vi "MTConnect_data.vi"() -> ()   [LabVIEW 2014]
panel:
  in  "Boolean":bool
  out "size(s)":i32
  out "Array":i32[](array[numeric])
  out "x-y":u32
  in  "Stop Program":bool
  out "CNC Machine":bool
  in  "?":enum32{""}(tab)
  out "Tool position Y":dbl[](graph)
  out "Spindle Speed":dbl[](graph)
  out "Tool position X":dbl[](graph)
  in  "Record speed":bool
  out "Feed rate":dbl[](graph)
  in  "Record feed ratre":bool
  in  "Record linear X":bool
  in  "Record linear Y":bool
  out "Machine status":string
  out "Program name":string
  out "Block of code being executed":string
  out "Machine availability":string
  out "Emergency status":string
  out "Controller mode":string
  in  "Record spindle \n      load":bool
  out "Spindle load":dbl[](graph)
  out "Spindle power consumption":dbl[](graph)
  in  "Record spindle  \n        power":bool
  in  "Record linear Z":bool
  out "Tool position Z":dbl[](graph)
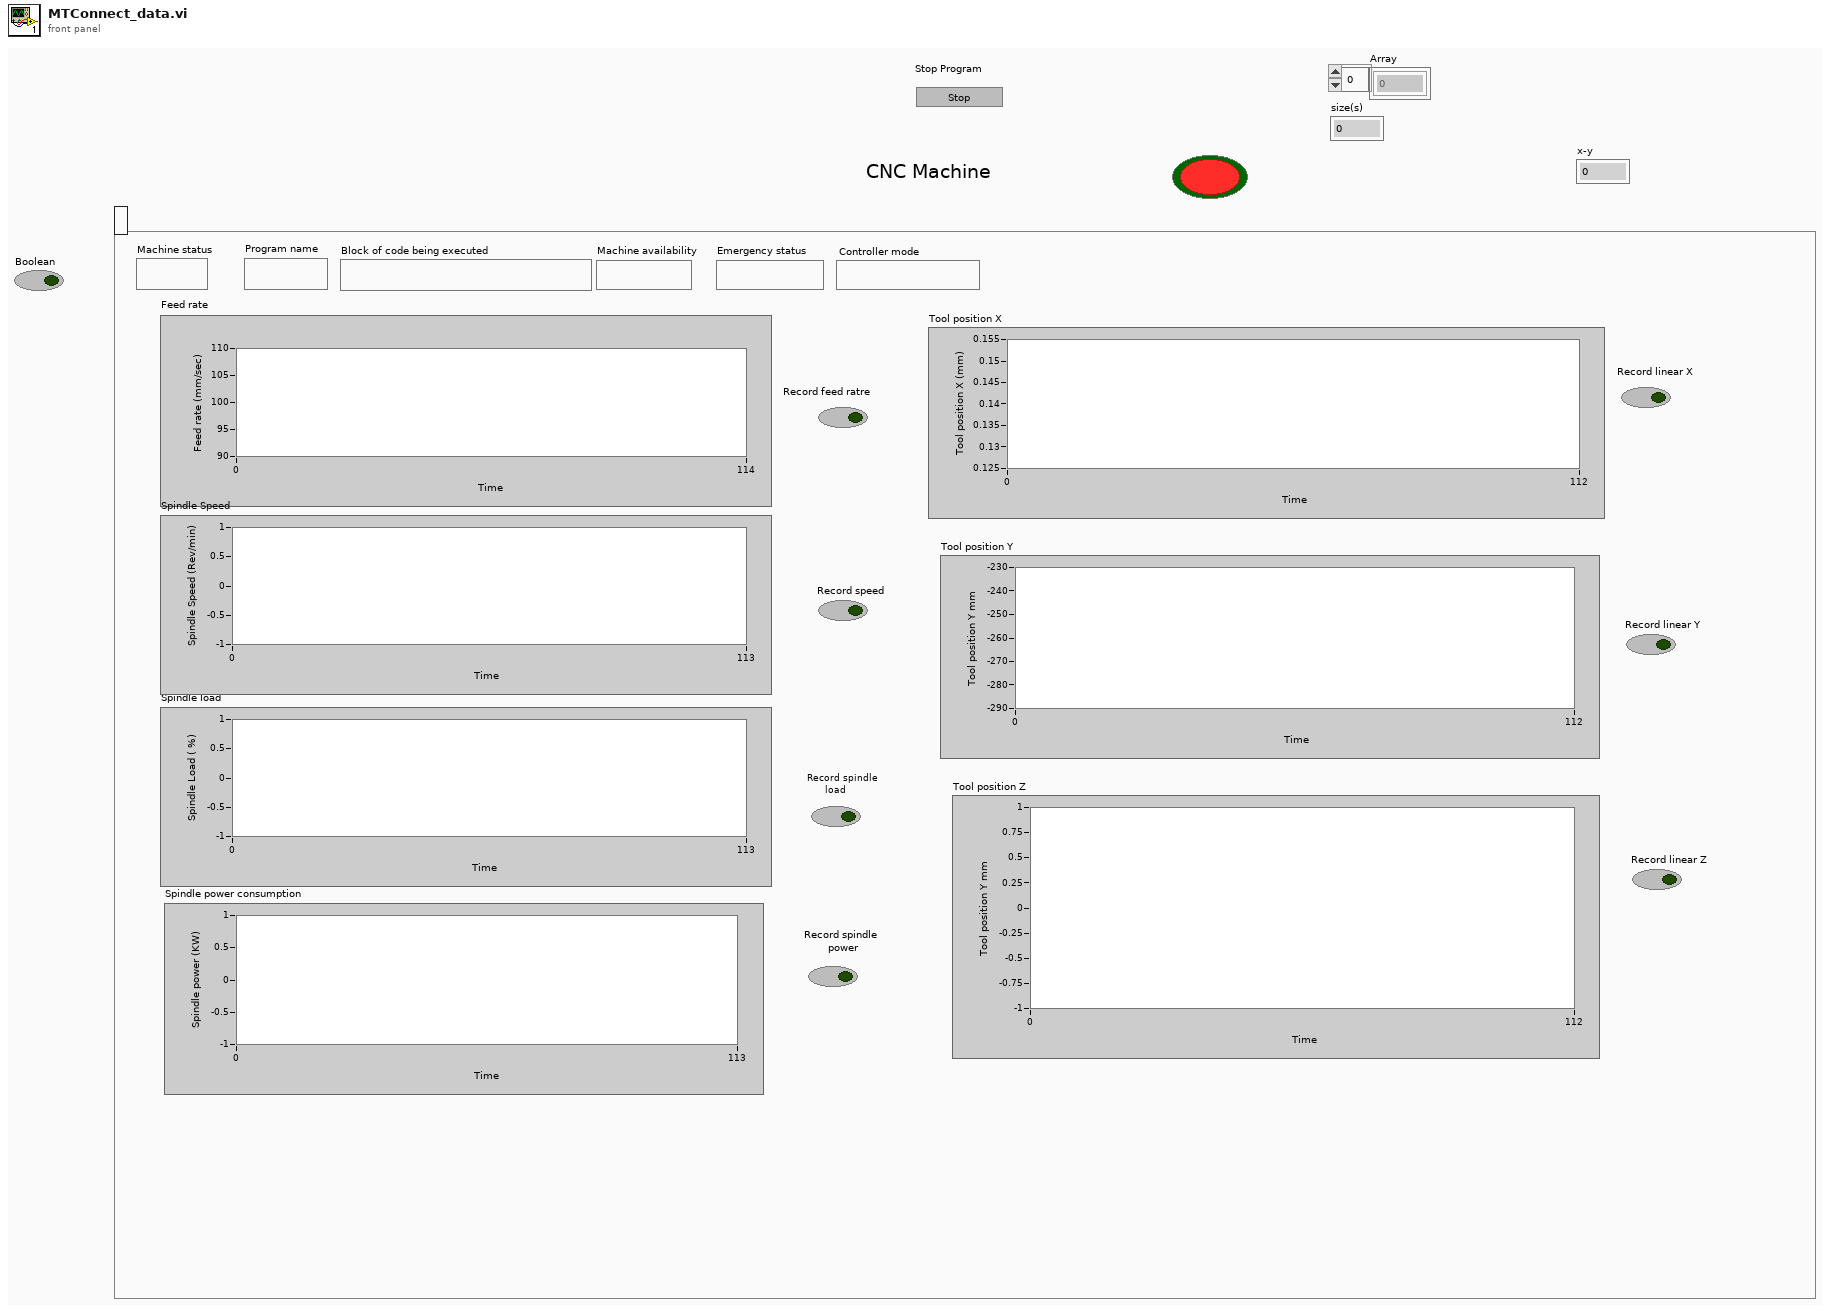
[diagram p1: front panel]
types:
  T1 = cluster{"Program status":string, "Bolck of code being executed":string, "Program name":string, "number":dbl[], "number":dbl[], "number":dbl[], "Boolean":bool}
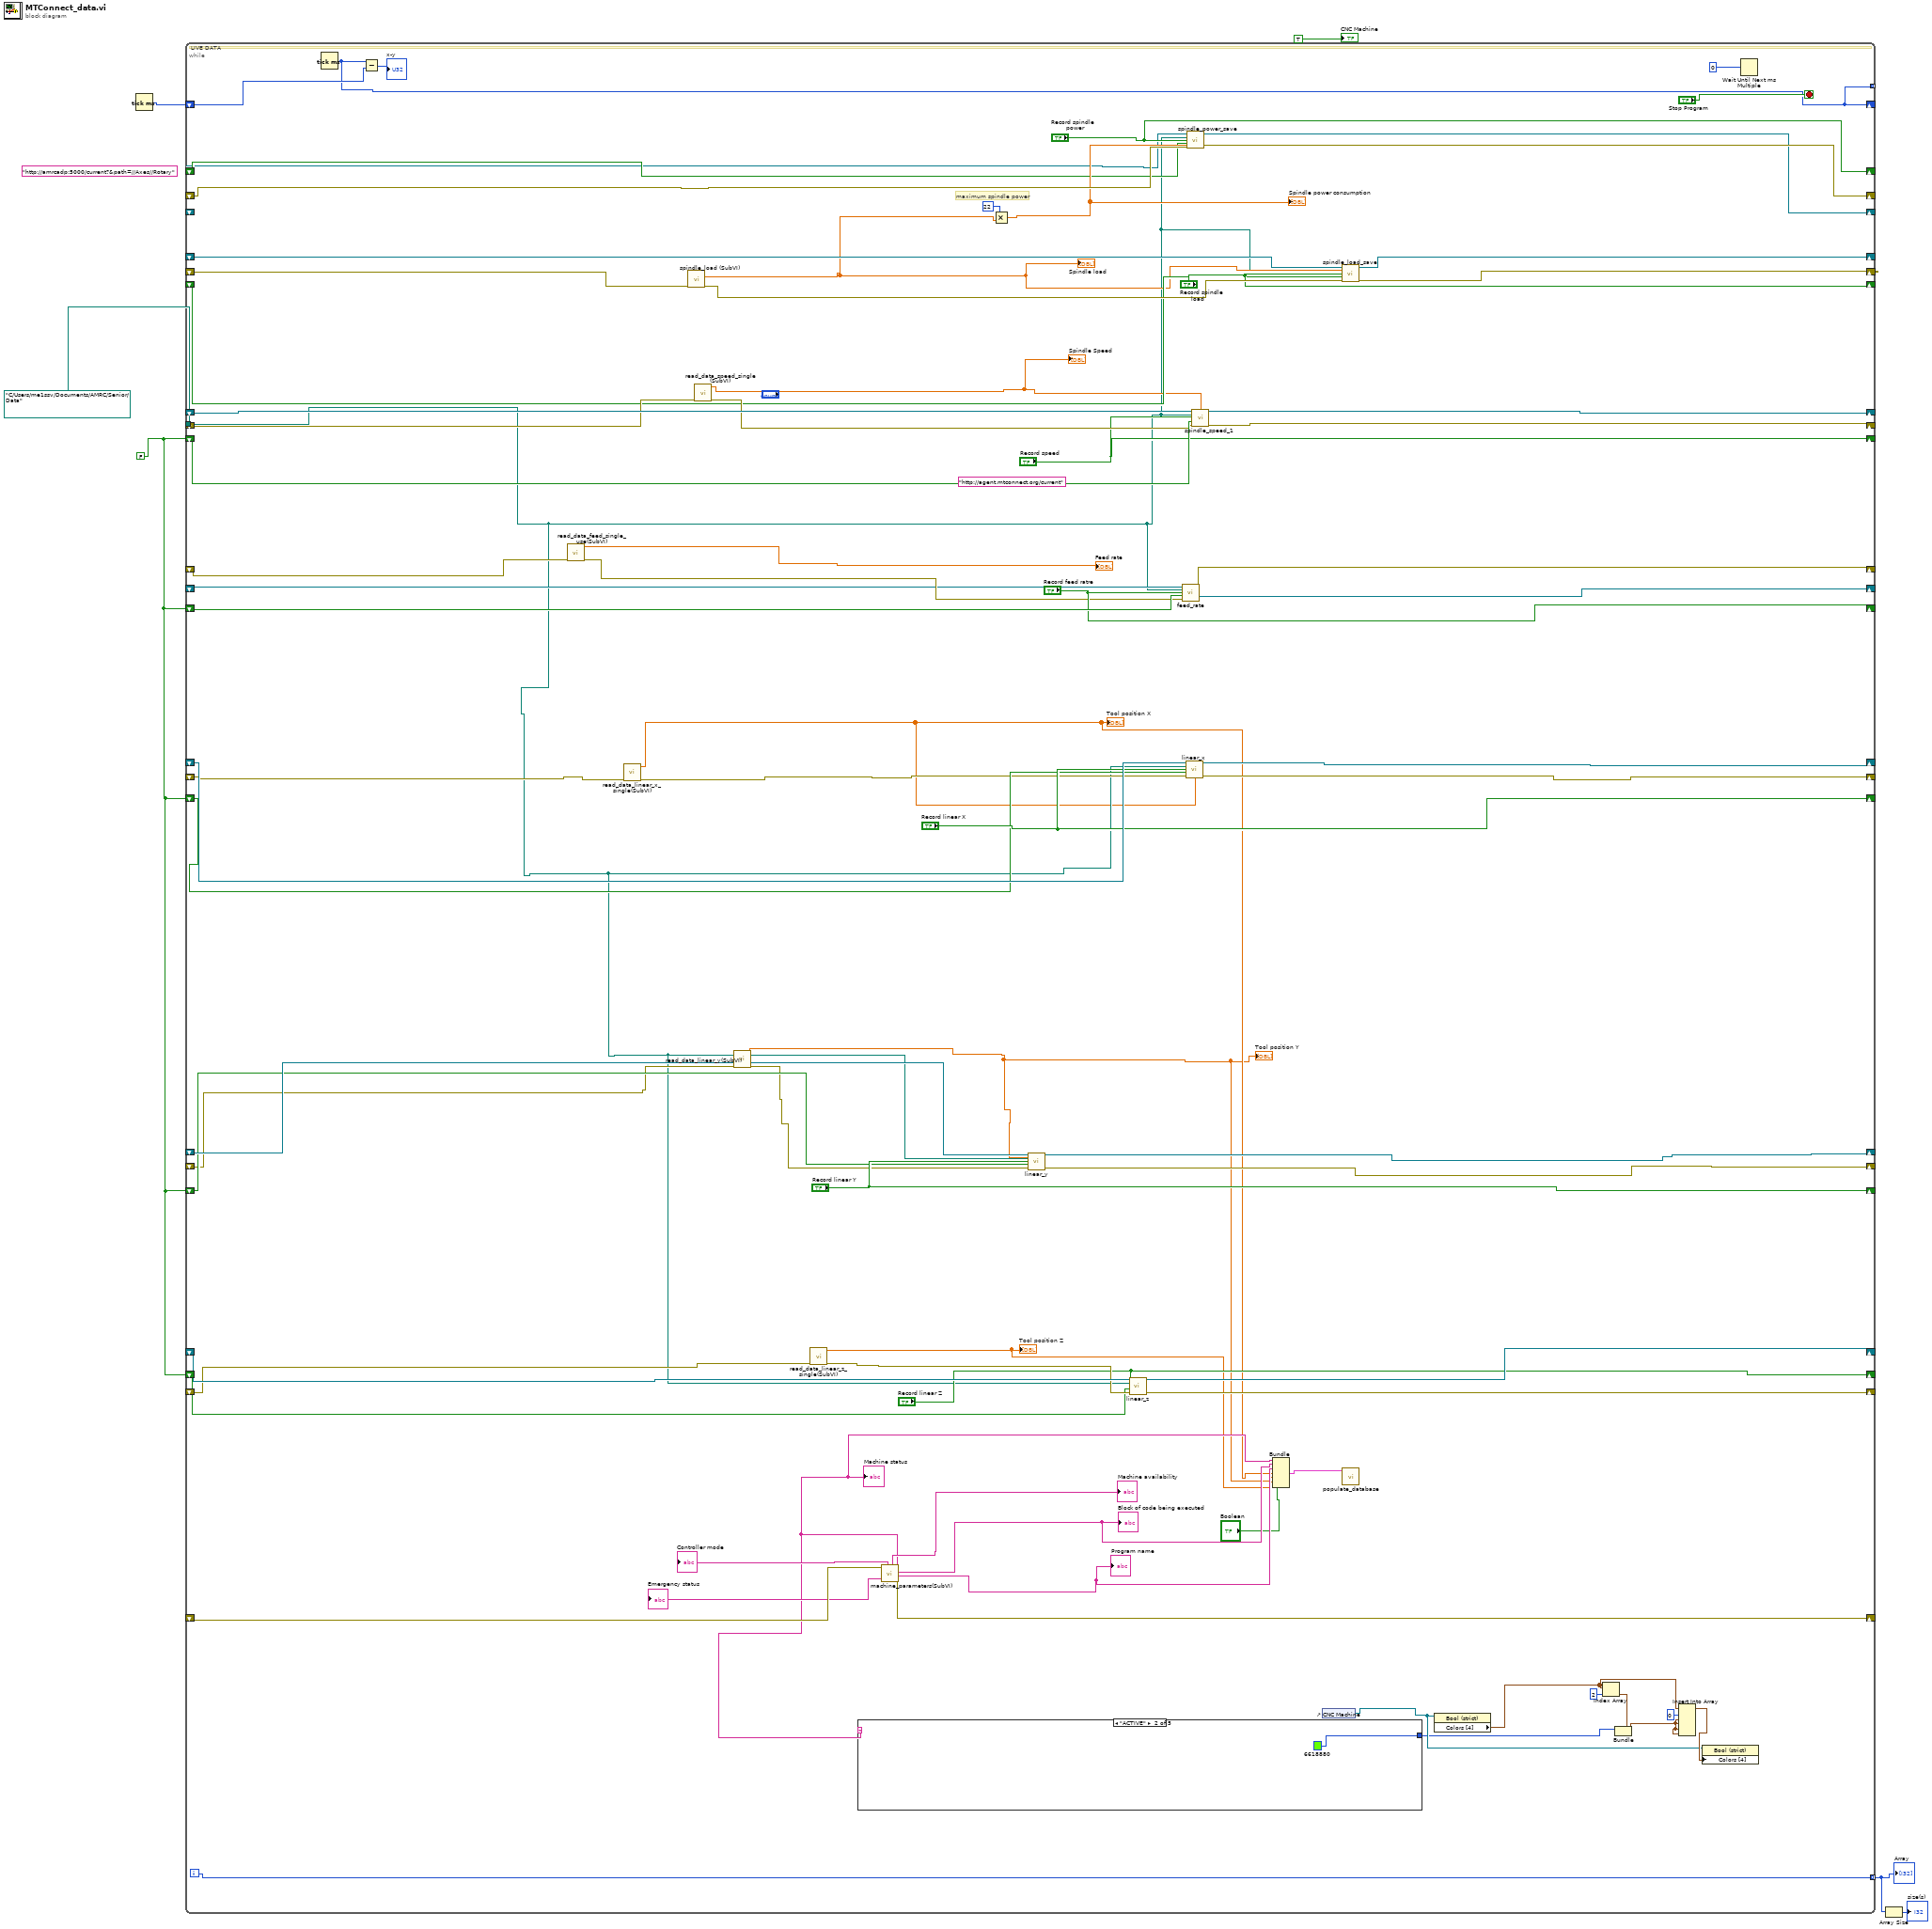
[diagram p0: block diagram]
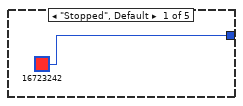
[diagram p2: hidden frame]
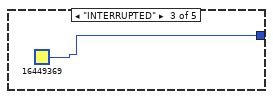
[diagram p3: hidden frame]
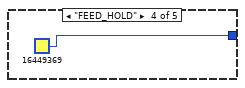
[diagram p4: hidden frame]
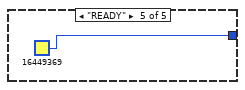
[diagram p5: hidden frame]
diagram:
  (unwired) "http://amrcadp:5000/current?&path=//Axes//Rotary" ("URL")
  w6 = FALSE ("Boolean 2")
  (unwired) "http://agent.mtconnect.org/current" ("URL")
  n1 = Tick Count (ms)() -> (millisecond timer value=w3:u32)
  n2 = while {
    shift-right: [w85] -> _
    shift-left: _ -> [w42]
    shift-right: ["Record speed"] -> _
    shift-left: w6 -> [w84]
    shift-right: [w87] -> _
    shift-left: _ -> [w86]
    shift-right: [w81] -> _
    shift-left: _ -> [w41]
    shift-right: ["Record feed ratre"] -> _
    shift-left: w6 -> [w83]
    shift-right: [w80] -> _
    shift-left: _ -> [w55]
    shift-right: [w75] -> _
    shift-left: _ -> [w53]
    shift-right: [w76] -> _
    shift-left: _ -> [w79]
    shift-right: ["Record linear X"] -> _
    shift-left: w6 -> [w77]
    shift-right: [w71] -> _
    shift-left: _ -> [w51]
    shift-right: ["Record linear Y"] -> _
    shift-left: w6 -> [w72]
    shift-right: [w70] -> _
    shift-left: _ -> [w74]
    shift-right: [w69] -> _
    shift-left: _ -> [w68]
    shift-right: [w67] -> _
    shift-left: _ -> [w50]
    shift-right: ["Record linear Z"] -> _
    shift-left: w6 -> [w19]
    shift-right: [w66] -> _
    shift-left: _ -> [w65]
    shift-right: [w38] -> _
    shift-left: _ -> [w40]
    shift-right: [w37] -> _
    shift-left: _ -> [w35]
    shift-right: [w32] -> _
    shift-left: _ -> [w23]
    shift-right: [w36] -> _
    shift-left: _ -> [w33]
    shift-right: ["Record spindle \n      load"] -> _
    shift-left: _ -> [w27]
    shift-right: ["Record spindle  \n        power"] -> _
    shift-left: _ -> [w25]
    tunnel: path "C:/Users/me1ssv/Documents/AMRC/Senior/Data" ("base path") -> [w20]
    shift-right: [w16] -> _
    shift-left: w3 -> [w18]
    tunnel: [w16] -> _ mode=indexing
    tunnel: [w15] -> w2 mode=indexing
    i -> [w15]
    stop <- "Stop Program" stop-if-true
    # "maximum spindle power"
    # "LIVE DATA"
    n3 = Tick Count (ms)() -> (millisecond timer value=w16:u32)
    n4 = Subtract(x=w16, y=w18) -> (x-y=→"x-y":u32)
    n5 = call "read_data_feed_single_use(SubVI).vi"("error in (no error)"=w55) -> ("error out"=w54:errorcluster, "appended array"=→"Feed rate":dbl[])  [unwired: 9 in]
    n6 = call "read_data_linear_x_single(SubVI).vi"("error in (no error)"=w53) -> ("error out"=w52:errorcluster, "number"=w11:dbl[])  [unwired: 9 in]
    "Tool position X" <- w11
    n7 = call "spindle_load (SubVI).vi"("error in (no error)"=w40) -> ("error out"=w39:errorcluster, "number"=w24:dbl[])  [unwired: 9 in]
    "Spindle load" <- w24
    n8 = call "read_data_speed_single (SubVI).vi"("error in (no error)"=w42) -> ("error out"=w56:errorcluster, "number"=w22:dbl[])  [unwired: 9 in]
    "Spindle Speed" <- w22
    n9 = call "read_data_linear_y(SubVI).vi"("error in (no error)"=w51) -> ("error out"=w48:errorcluster, "number"=w10:dbl[])  [unwired: 9 in]
    "Tool position Y" <- w10
    n10 = call "read_data_linear_z_single(SubVI).vi"("error in (no error)"=w50) -> ("error out"=w49:errorcluster, "number"=w9:dbl[])  [unwired: 9 in]
    "Tool position Z" <- w9
    n11 = call "machine_parameters(SubVI).vi"("error in (no error) 3"=w65) -> ("error out 3"=w66:errorcluster, "Program name"=w12:string, "Bolck of code being executed"=w13:string, "Program status"=w14:string, "Machine availability"=→"Machine availability":string, "Emergency status"=→"Emergency status":string, "Controller mode"=→"Controller mode":string)  [unwired: 3 in, 1 out]
    "Machine status" <- w14
    "Program name" <- w12
    "Block of code being executed" <- w13
    n12 = case shown="\"ACTIVE\"" w14 {
      tunnel: [u32 16723242 u32 6618880 u32 16449369 u32 16449369 u32 16449369] -> w57
      frame "Stopped", Default {
      }
      frame "ACTIVE" {
      }
      frame "INTERRUPTED" {
      }
      frame "FEED_HOLD" {
      }
      frame "READY" {
      }
    }
    n13 = Multiply(x=22, y=w24) -> (x*y=w30:dbl[])
    "Spindle power consumption" <- w30
    n14 = call "linear_y.vi"("Byte Stream File in"=w74, "Array"=w10, "base path"=w20, "Record  SS 661"="Record linear Y", "Boolean 3"=w72, "error in (no error)"=w48) -> ("Byte Stream File out"=w70:refnum<file>, "error out"=w71:errorcluster)  [unwired: 5 in, 3 out]
    n15 = call "linear_z.vi"("Byte Stream File in"=w68, "base path"=w20, "Record  SS 661"="Record linear Z", "Boolean 3"=w19, "error in (no error)"=w49) -> ("Byte Stream File out"=w69:refnum<file>, "error out"=w67:errorcluster)  [unwired: 6 in, 3 out]
    n16 = call "feed_rate.vi"("Byte Stream File in"=w41, "base path"=w20, "Record  SS 661"="Record feed ratre", "Boolean 3"=w83, "error in (no error)"=w54) -> ("Byte Stream File out"=w81:refnum<file>, "error out"=w80:errorcluster)  [unwired: 6 in, 3 out]
    n17 = call "linear_x.vi"("Byte Stream File in"=w79, "Array"=w11, "base path"=w20, "Record  SS 661"="Record linear X", "Boolean 3"=w77, "error in (no error)"=w52) -> ("Byte Stream File out"=w76:refnum<file>, "error out"=w75:errorcluster)  [unwired: 5 in, 3 out]
    n18 = call "spindle_power_save.vi"("Byte Stream File in"=w23, "Array"=w30, "base path"=w20, "Record  SS 661"="Record spindle  \n        power", "Boolean 3"=w25, "error in (no error)"=w33) -> ("Byte Stream File out"=w32:refnum<file>, "error out"=w36:errorcluster)  [unwired: 7 in, 1 out]
    n19 = call "spindle_speed_1.vi"("Byte Stream File in"=w86, "Array"=w22, "base path"=w20, "Record  SS 661"="Record speed", "Boolean 3"=w84, "error in (no error)"=w56) -> ("Byte Stream File out"=w87:refnum<file>, "error out"=w85:errorcluster)  [unwired: 5 in, 3 out]
    n20 = Bundle("Program status"=w14, "Bolck of code being executed"=w13, "Program name"=w12, "number"=w11, "number"=w10, "number"=w9, "Boolean"="Boolean") -> (w7:T1)  [unwired: 1 in]
    n21 = control-ref of="CNC Machine"() -> (w58:refnum<vi>)
    n22 = call "spindle_load_save.vi"("Byte Stream File in"=w35, "Array"=w24, "base path"=w20, "Record  SS 661"="Record spindle \n      load", "Boolean 3"=w27, "error in (no error)"=w39) -> ("Byte Stream File out"=w37:refnum<file>, "error out"=w38:errorcluster)  [unwired: 5 in, 3 out]
    n23 = call "populate_database.vi"("output cluster"=w7) -> ()  [unwired: 11 in]
    n24 = property on="Property Node" class="Bool (strict)"(reference=w58) -> ("Colors [4]"=w59:cluster{u32, u32}[])  [unwired: 1 in, 2 out]
    n25 = Index Array(array=w59, index=2) -> (element=w61:cluster{u32, u32})
    n26 = Bundle(cluster=w61, w57) -> (w62:cluster{u32, u32})  [unwired: 1 in]
    n27 = Insert Into Array(array=w59, index=0, new element #1=w62, new element #2=w62, new element #3=w62, new element #4=w62) -> (w60:cluster{u32, u32}[])
    n28 = property on="Property Node" class="Bool (strict)"(reference=w58, "Colors [4]"=w60) -> ()  [unwired: 1 in, 2 out]
    n29 = Wait Until Next ms Multiple(millisecond multiple=u32 0) -> ()  [unwired: 1 out]
  }
  "Array" <- w2
  n30 = Array Size(array=w2) -> (size(s)=→"size(s)":i32)
  "CNC Machine" <- TRUE
